vi "_Read.vi"(8 "error in (no error)":errorcluster, 11 "Cryostat in":refnum<class "Cryostat.lvclass">) -> (0 "error out":errorcluster, 2 "array of two temperatures":dbl[](array[numeric]), 3 "Cryostat out":refnum<class "Cryostat.lvclass">)   [LabVIEW 2017, in "Cryostat.lvclass"]
doc: "(Protected, Dynamic, Pure Virtual/Abstract) Perform a measurement and return one or more channels of data. Outsiders should not call this method, but instead the public \"Read Data.vi\"."
uses:
  Cryostat.lvclass
  Cryostat.lvclass/Cryostat.ctl
  Utility Classes/Readable/Readable.lvclass
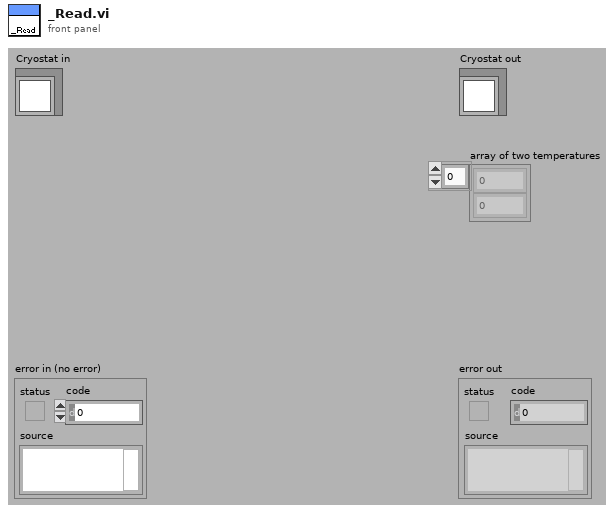
[diagram p1: front panel]
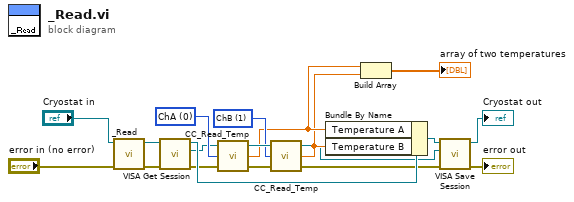
[diagram p0: block diagram]
diagram:
  w11 = u8 1 items=["ChA", "ChB", "ChC", "ChD"] ("Input")
  w12 = u8 0 items=["ChA", "ChB", "ChC", "ChD"] ("Input")
  n1 = call-parent "_Read.vi"("error in (no error)"="error in (no error)", "Readable in"="Cryostat in") -> ("error out"=w9:errorcluster, "Readable out"=w10:refnum<class "Cryostat.lvclass">)  [unwired: 7 in, 1 out]
  n2 = call-dynamic "VISA Get Session.vi"("error in (no error)"=w9, "Instrument.lvclass in"=w10) -> ("error out"=w15:errorcluster, "VISA Resource Name"=w4:refnum<visa-resource-name>, "Instrument.lvclass out"=w17:refnum<class "Cryostat.lvclass">)  [unwired: 7 out]
  n3 = call "CC_Read_Temp.vi"("error in (no error)"=w15, "Input"=w12, "VISA In"=w4) -> ("error out"=w14:errorcluster, "Temperature"=w8:dbl, "VISA Out"=w13:refnum<visa-resource-name>)
  n4 = call "CC_Read_Temp.vi"("error in (no error)"=w14, "Input"=w11, "VISA In"=w13) -> ("error out"=w2:errorcluster, "Temperature"=w7:dbl, "VISA Out"=w3:refnum<visa-resource-name>)
  n5 = Bundle By Name(cluster=w17, "Temperature A"=w8, "Temperature B"=w7) -> (w16:refnum<class "Cryostat.lvclass">)
  n6 = Build Array(w8, w7) -> (→"array of two temperatures":dbl[])
  n7 = call-dynamic "VISA Save Session.vi"("error in (no error)"=w2, "VISA Resource Name"=w3, "Instrument.lvclass in"=w16) -> ("error out"=→"error out":errorcluster, "Instrument.lvclass out"=→"Cryostat out":refnum<class "Cryostat.lvclass">)  [unwired: 7 out]
